vi "Inter2Line.vi"(9 "Length":u32, 10 "Scaling(dist/pix)":dbl, 11 "Intersections":T1[](array[typedef])) -> (3 "FilledLine":u32[](array[numeric]))   [LabVIEW 2014]
uses:
  TypeDefs/Point2DwSlope.ctl
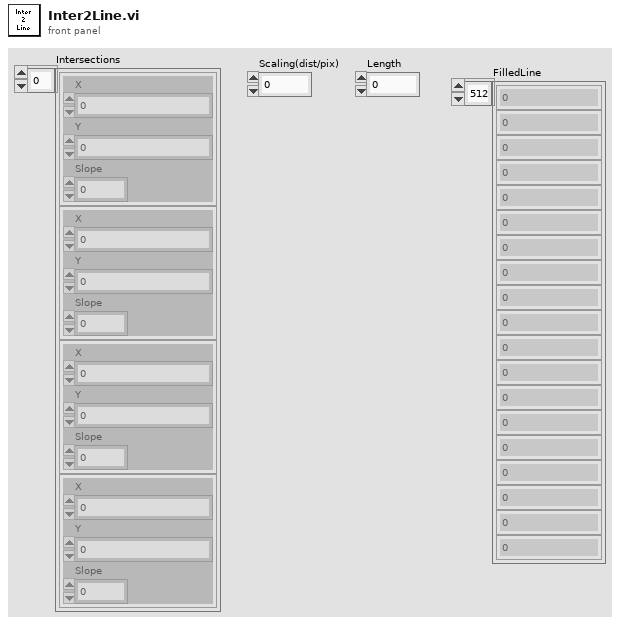
[diagram p1: front panel]
types:
  T1 = typedef "Point2DwSlope.ctl" = cluster{"X":sgl, "Y":sgl, "Slope":dbl}
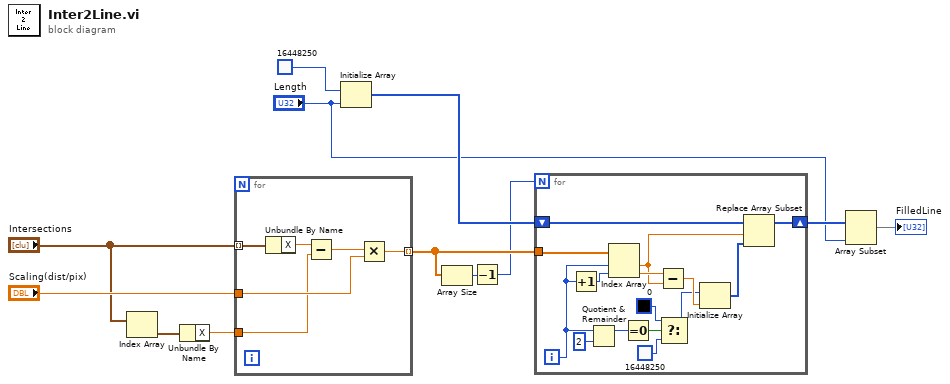
[diagram p0: block diagram]
diagram:
  n1 = Index Array(array="Intersections") -> (element=w10:T1)  [unwired: 1 in]
  n2 = Unbundle By Name(w10) -> ("X"=w9:sgl)
  n3 = for {
    tunnel: "Intersections" -> [w18] mode=indexing
    tunnel: "Scaling(dist/pix)" -> [w17]
    tunnel: [w13] -> w7 mode=indexing
    tunnel: w9 -> [w15]
    n4 = Unbundle By Name(w18) -> ("X"=w16:sgl)
    n5 = Subtract(x=w16, y=w15) -> (x-y=w14:sgl)
    n6 = Multiply(x=w14, y=w17) -> (x*y=w13:dbl)
  }
  n7 = Initialize Array(u32 16448250, "Length") -> (w8:u32[])
  n8 = Array Size(array=w7) -> (size(s)=w6:i32)
  n9 = Decrement(x=w6) -> (x-1=w5:i32)
  n10 = for {
    N: w5 -> [_]
    tunnel: w7 -> [w32]
    shift-right: [w23] -> w3
    shift-left: w8 -> [w33]
    i -> [w30]
    n11 = Increment(x=w30) -> (x+1=w31:i32)
    n12 = Quotient & Remainder(x=w30, y=2) -> (x-y*floor(x/y)=w28:i32)  [unwired: 1 out]
    n13 = Index Array(array=w32, index #1=w30, index #2=w31) -> (element #1=w19:dbl, element #2=w20:dbl)
    n14 = Equal To 0?(x=w28) -> (x = 0?=w27:bool)
    n15 = Subtract(x=w20, y=w19) -> (x-y=w22:dbl)
    n16 = Select(t=u32 0, s=w27, f=u32 16448250) -> (s? t:f=w21:u32)
    n17 = Initialize Array(w21, w22) -> (w24:u32[])
    n18 = Replace Array Subset(array=w33, new element=w24, index=w19) -> (w23:u32[])
  }
  n19 = Array Subset(array=w3, length="Length") -> (→"FilledLine":u32[])  [unwired: 1 in]
